vi "AVI to TIFF (Folder).vi"() -> ()   [LabVIEW 2012]
panel:
  in  "Folder":path
  in  "Delete AVI?":bool
  out "error out":errorcluster
  in  "Error in (no error)":errorcluster
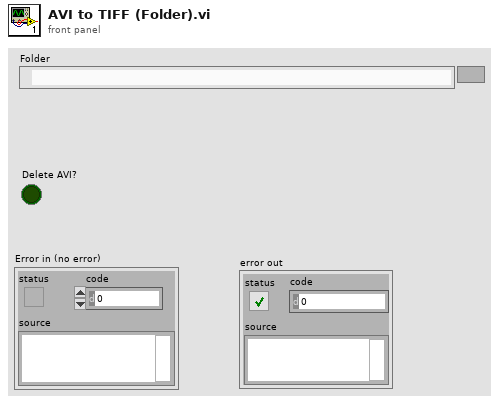
[diagram p1: front panel]
types:
  T1 = typedef "IMAQ Image.ctl" = refnum<image>
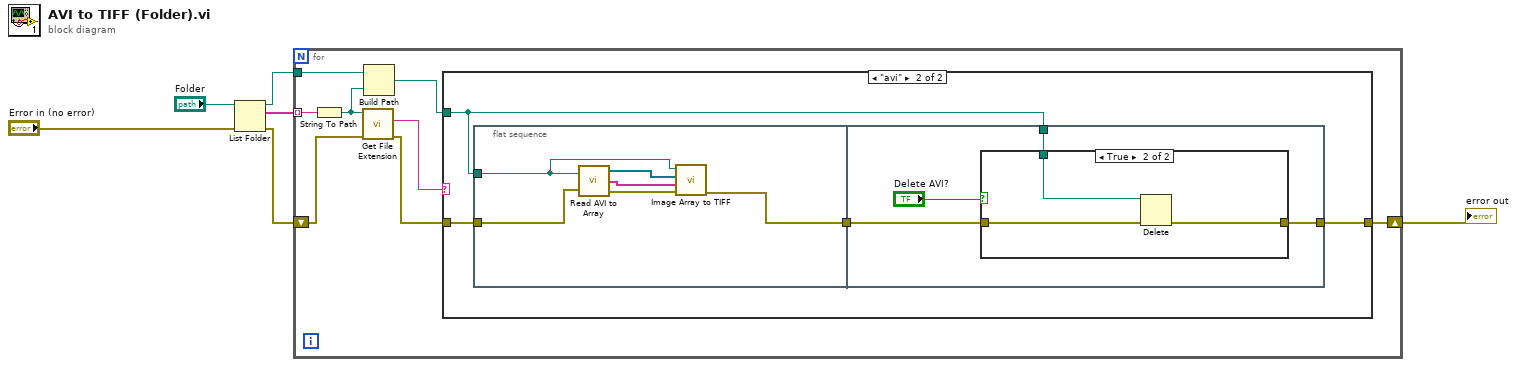
[diagram p0: block diagram]
diagram:
  n1 = List Folder(path="Folder", error in="Error in (no error)") -> (path out=w1:path, filenames=w5:string[], error out=w3:errorcluster)  [unwired: 2 in, 1 out]
  n2 = for {
    shift-right: [w14] -> w6
    shift-left: w3 -> [w11]
    tunnel: w5 -> [w13] mode=indexing
    tunnel: w1 -> [w9]
    n3 = String To Path(string=w13) -> (path=w8:path)
    n4 = call <vilib>:"Get File Extension.vi"("error in (no error)"=w11, "file"=w8) -> ("error out"=w12:errorcluster, "lowercase file extension"=w10:string)  [unwired: 6 in, 2 out]
    n5 = Build Path(base path=w9, name or relative path=w8) -> (appended path=w7:path)
    n6 = case shown="\"avi\"" w10 {
      tunnel: [w15 w18] -> w14
      tunnel: w12 -> [w15 w17]
      tunnel: w7 -> [_ w16]
      frame Default {
      }
      frame "avi" {
        n7 = flat-sequence {
          tunnel: [w22] -> w19
          tunnel: w17 -> [w21]
          tunnel: w16 -> [w20]
          tunnel: w19 -> [w28]
          tunnel: [w27] -> w18
          tunnel: w16 -> [w26]
          frame #0 {
            n8 = call "Read AVI to Array.vi"("AVI Path"=w20, "Error in (no error)"=w21) -> ("Image Array"=w25:T1[], "Data Array"=w24:string[], "Error out"=w23:errorcluster)
            n9 = call "Image Array to TIFF.vi"("error in"=w23, "Data Array"=w24, "Image Array"=w25, "Destination Image File"=w20) -> ("error out"=w22:errorcluster)  [unwired: 7 in]
          }
          frame #1 {
            n10 = case shown="True" "Delete AVI?" {
              tunnel: w28 -> [w30 w33]
              tunnel: [w30 w32] -> w27
              tunnel: w26 -> [_ w31]
              frame False {
              }
              frame True {
                n11 = Delete(path (use dialog)=w31, error in=w33) -> (error out=w32:errorcluster)  [unwired: 3 in, 2 out]
              }
            }
          }
        }
      }
    }
  }
  "error out" <- w6
